vi "Actor Core.vi"(8 "error in":errorcluster, 11 "ResultsViewer in":refnum<class "ResultsViewer.lvclass">) -> (0 "error out":errorcluster, 3 "Actor out":refnum<class "Actor.lvclass">)   [LabVIEW 2019, in "ResultsViewer.lvlib" / "ResultsViewer.lvclass"]
doc: "(<B>Filename</B>: Actor Framework.lvlib:Actor.lvclass:Actor Core.vi)\n\nReceives messages to the actor, reacts to them, and initiates any error handling that may shut the actor down.\n\nDescendant classes may override this VI to append parallel tasks for the actor to complete while it handles messages. Overrides use the Call Parent Class Method node."
uses:
  ResultsViewer.lvclass
  C:/Program Files (x86)/National Instruments/LabVIEW 2019/vi.lib/ActorFramework/Actor/Actor.lvclass
  <vilib>/ActorFramework/Actor/Actor.lvclass
  ResultsViewer.lvclass/ResultsViewer.ctl
  <vilib>/ActorFramework/Actor/Actor.lvclass/Actor.ctl
  <vilib>/ActorFramework/Message Enqueuer/Message Enqueuer.lvclass/Message Enqueuer.ctl
  <vilib>/ActorFramework/Message Enqueuer/Init from Existing Queue.vi
  <vilib>/ActorFramework/Message Enqueuer/Enqueue.vi
  <vilib>/ActorFramework/Stop Msg/Stop Msg.lvclass
  C:/Program Files (x86)/National Instruments/LabVIEW 2019/vi.lib/ActorFramework/Message/Message.lvclass
  <vilib>/ActorFramework/Message Priority Queue/Priority Enqueue.vi
  <vilib>/ActorFramework/Message Enqueuer/Message Enqueuer.lvclass
panel:
  out "Loaded TDMS Filename":string
  out "O2 Saturation":dbl[](graph)
  out "Heart beat":dbl[](graph)
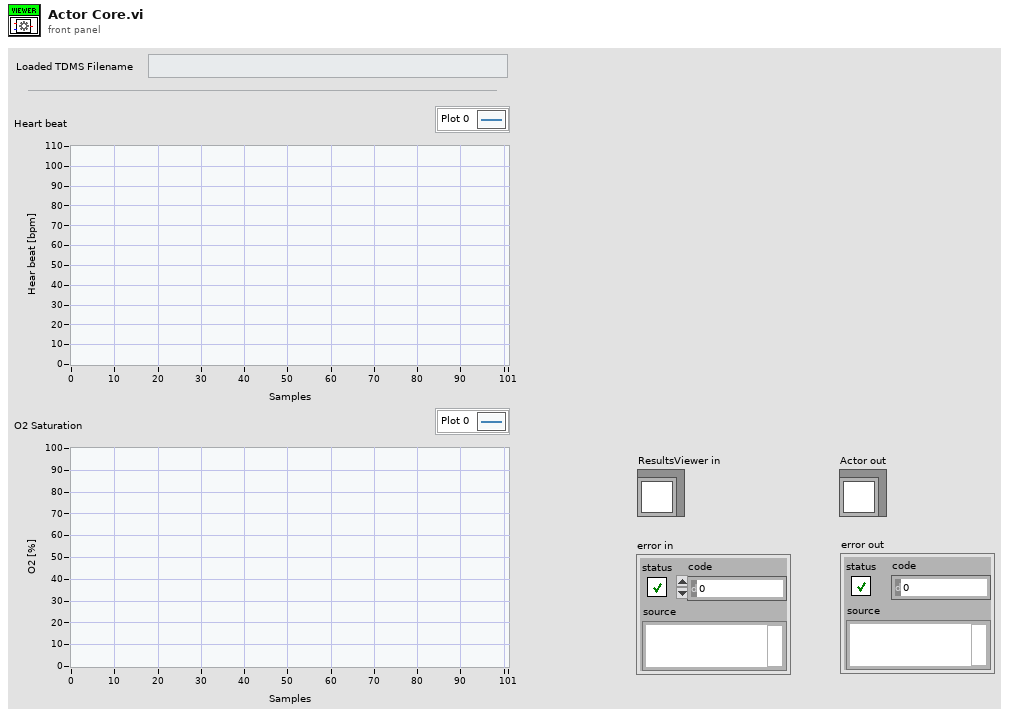
[diagram p1: front panel]
types:
  T1 = enum32{"Invalid", "Standard", "Closed", "Hidden", "Minimized", "Maximized"}
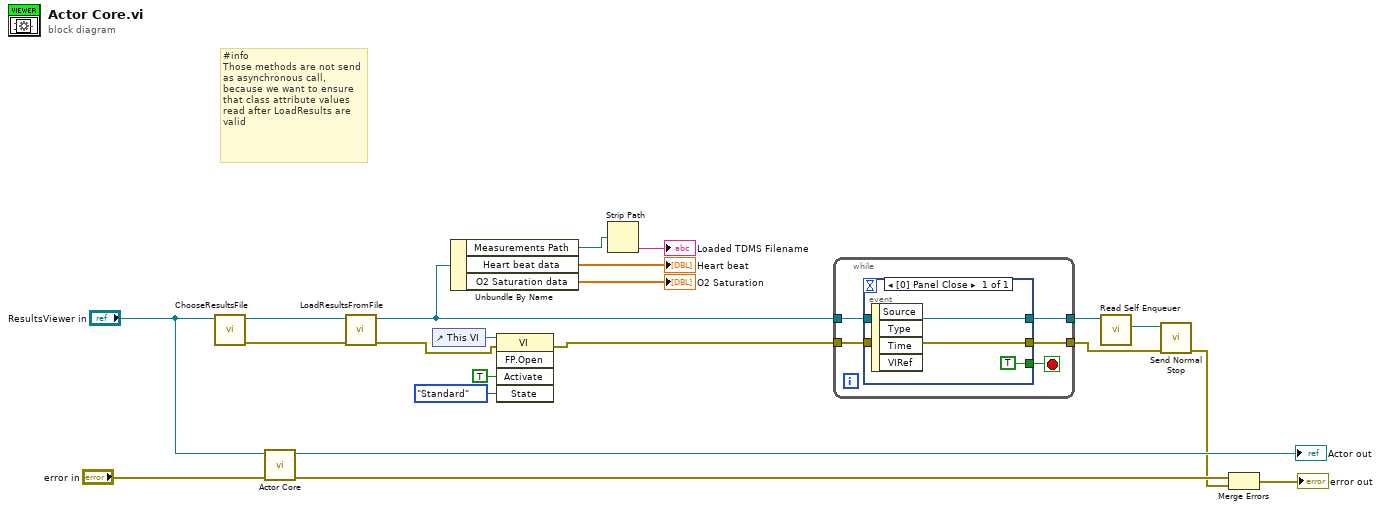
[diagram p0: block diagram]
diagram:
  # "#info\nThose methods are not send as asynchronous call, because we want to ensure that class attribute values read after LoadResults are valid"
  n1 = call "ChooseResultsFile.vi"("ResultsViewer in"="ResultsViewer in") -> ("error out"=w16:errorcluster, "ResultsViewer out"=w17:refnum<class "ResultsViewer.lvclass">)  [unwired: 8 in, 1 out]
  n2 = call-parent "Actor Core.vi"("error in"="error in", "Actor in"="ResultsViewer in") -> ("error out"=w21:errorcluster, "Actor out"=→"Actor out":refnum<class "Actor.lvclass">)  [unwired: 8 in]
  n3 = call "LoadResultsFromFile.vi"("error in (no error)"=w16, "ResultsViewer in"=w17) -> ("error out"=w3:errorcluster, "ResultsViewer out"=w11:refnum<class "ResultsViewer.lvclass">)  [unwired: 8 in]
  n4 = control-ref of="This VI"() -> (w6:refnum<vi>)
  n5 = Unbundle By Name(w11) -> ("Measurements Path"=w8:path, "Heart beat data"=→"Heart beat":dbl[], "O2 Saturation data"=→"O2 Saturation":dbl[])
  n6 = invoke class="VI" method="FP.Open"(reference=w6, error in=w3, "Activate"=TRUE ("Activate?"), "State"=T1."Standard") -> (error out=w2:errorcluster)  [unwired: 1 in, 4 out]
  n7 = Strip Path(path=w8) -> (name=→"Loaded TDMS Filename":string)  [unwired: 1 out]
  n8 = while {
    tunnel: w2 -> [w25]
    tunnel: w11 -> [w26]
    tunnel: [w24] -> w1
    tunnel: [w23] -> w14
    stop <- w22 stop-if-true
    n9 = event shown="[0] Panel Close" {
      selector: _ -> [_]
      dyn-events: _ -> [_]
      timeout: _ -> [_]
      tunnel: w26 -> [w28]
      tunnel: w25 -> [w29]
      tunnel: [w29] -> w24
      tunnel: [w28] -> w23
      tunnel: [TRUE] -> w22
      event Panel Close {
        n10 = event-data() -> ()  [unwired: 1 in, 4 out]
      }
    }
  }
  n11 = call <vilib>:"Read Self Enqueuer.vi"("Actor"=w14) -> ("Self Enqueuer"=w12:refnum<class "Message Enqueuer.lvclass">)  [unwired: 10 in]
  n12 = call <vilib>:"Send Normal Stop.vi"("error in (no error)"=w1, "Message Enqueuer"=w12) -> ("error out"=w13:errorcluster)  [unwired: 9 in]
  n13 = Merge Errors(w21, w13) -> (→"error out":errorcluster)
